vi "PID Integral Control.vi"(0 "Temp In (deg C)":dbl format="%.2f", 2 "in control band":bool, 7 "Control Parameters":T1={"Setpoint"=50.0, "Control Bandwidth"=4.0, "Integral Time"=30.0, "Int\nON"=TRUE, "Derivative Tme"=0.5, "Der\nON"=TRUE, "Settle Bandwidth"=1.0, "Settle Time"=200.0} {"Settle Time" step=1.0; "Settle Bandwidth" step=0.01; "Derivative Tme" step=0.01; "Integral Time" step=1.0; "Control Bandwidth" step=0.1; "Setpoint" step=0.1}, 9 "reset":bool, 11 "delta t":dbl format="%.2f") -> (8 "Integral Power":dbl format="%.2f")   [LabVIEW 2019]
doc: "This is a Bug C(T) subVI.\n\nThis VI does the PID integral calculation.\n\nIt zeroes the integral power on INT off, startup, reset, or after experiencing two temperature measurements in a row outside of the control band.\n\nPaul K Dixon\nPhysics 3600\nCSUSB Physics"
uses:
  typedefs/PID control parameters.ctl
panel:
  # "PID\nIntegral\nPower\nControl"
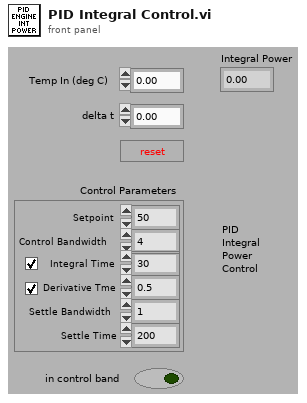
[diagram p1: front panel]
types:
  T1 = typedef "PID control parameters.ctl" = cluster{"Setpoint":dbl, "Control Bandwidth":dbl, "Integral Time":dbl, "Int\nON":bool, "Derivative Tme":dbl, "Der\nON":bool, "Settle Bandwidth":dbl, "Settle Time":dbl}
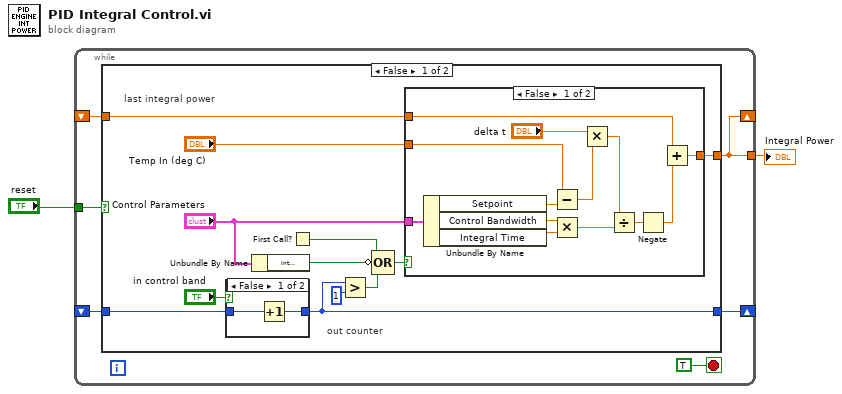
[diagram p0: block diagram]
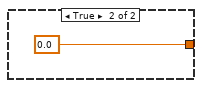
[diagram p2: hidden frame]
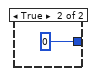
[diagram p3: hidden frame]
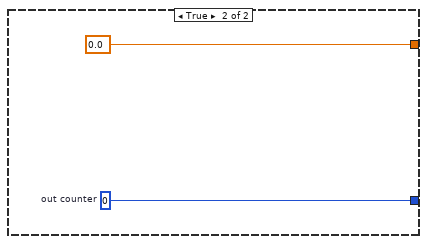
[diagram p4: hidden frame]
diagram:
  n1 = while {
    tunnel: [w3] -> w1
    tunnel: "reset" -> [w4]
    shift-left: _ -> [w5]
    shift-right: [w3] -> _
    shift-left: _ -> [w6]
    shift-right: [w7] -> _
    stop <- TRUE stop-if-true
    n2 = case shown="False" w4 {
      tunnel: [w16 0.0] -> w3
      tunnel: [w14 w38] -> w7
      tunnel: w6 -> [w13 _]
      tunnel: w5 -> [w12 _]
      frame False {
        # "out counter"
        # "last integral power"
        n3 = case shown="False" "in control band" {
          tunnel: w13 -> [w36 _]
          tunnel: [w35 u32 0] -> w14
          frame False {
            n4 = Increment(x=w36) -> (x+1=w35:u32)
          }
          frame True {
          }
        }
        n5 = Unbundle By Name("Control Parameters") -> ("Int\nON"=w10:bool)
        n6 = First Call?() -> (First Call?: T/F=w9:bool)
        n7 = Greater?(x=w14, y=u32 1) -> (0:w17:bool)
        n8 = Compound Arithmetic op=OR(w9, invert w10, w17) -> (w18:bool)
        n9 = case shown="False" w18 {
          tunnel: "Temp In (deg C)" -> [w33 _]
          tunnel: "Control Parameters" -> [w31 _]
          tunnel: w12 -> [w24 _]
          tunnel: [w22 0.0] -> w16
          frame False {
            n10 = Unbundle By Name(w31) -> ("Setpoint"=w32:dbl, "Control Bandwidth"=w30:dbl, "Integral Time"=w29:dbl)
            n11 = Subtract(x=w33, y=w32) -> (x-y=w28:dbl)
            n12 = Multiply(x=w30, y=w29) -> (x*y=w25:dbl)
            n13 = Multiply(x="delta t", y=w28) -> (x*y=w26:dbl)
            n14 = Divide(x=w26, y=w25) -> (x/y=w23:dbl)
            n15 = Negate(x=w23) -> (-x=w21:dbl)
            n16 = Add(x=w24, y=w21) -> (x+y=w22:dbl)
          }
          frame True {
          }
        }
      }
      frame True {
        w38 = u32 0  # out counter
      }
    }
  }
  "Integral Power" <- w1
